vi "ServerCommand.vi"(0 "Command":string) -> (1 "Error":bool, 2 "Reply":string)   [LabVIEW 2014]
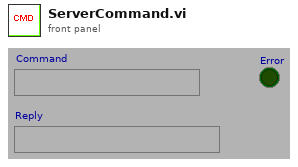
[diagram p1: front panel]
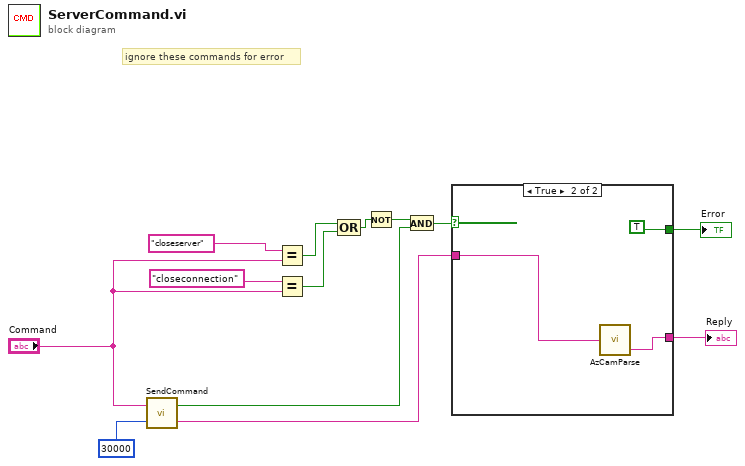
[diagram p0: block diagram]
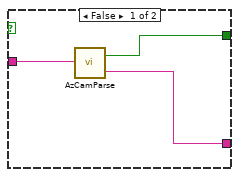
[diagram p2: hidden frame]
diagram:
  # "ignore these commands for error"
  n1 = call "SendCommand.vi"("timeout ms"=30000, "command"="Command") -> ("reply"=w10:string, "Error"=w6:bool)
  n2 = Equal?(x="closeserver" ("y"), y="Command") -> (x = y?=w2:bool)
  n3 = Equal?(x="closeconnection" ("y"), y="Command") -> (x = y?=w1:bool)
  n4 = Compound Arithmetic op=OR(w2, w1) -> (w12:bool)
  n5 = Not(x=w12) -> (.not. x?=w9:bool)
  n6 = And(x=w9, y=w6) -> (x .and. y?=w7:bool)
  n7 = case shown="True" w7 {
    tunnel: w10 -> [w16 w17]
    tunnel: [w15 TRUE ("Error")] -> w5
    tunnel: [w14 w18] -> w4
    frame False {
      n8 = call "AzCamParse.vi"("InputString"=w16) -> ("Error"=w15:bool, "Reply"=w14:string)
    }
    frame True {
      n9 = call "AzCamParse.vi"("InputString"=w17) -> ("Reply"=w18:string)  [unwired: 1 out]
    }
  }
  "Reply" <- w4
  "Error" <- w5
